vi "User_Database_Open.vi"(8 "error in (no error)":errorcluster caption="错误输入（无错误）", 11 "db Path":path=path "G:/2023项目/陆译电子/0008 User Management/Config/User_Info/User_Info.db") -> (0 "error out":errorcluster caption="错误输出", 3 "SQLite Connection":refnum<class "Connection.lvclass">)   [LabVIEW 2020]
uses:
  <vilib>/drjdpowell/SQLite Library/SQL Connection/Connection.lvclass
  <vilib>/drjdpowell/SQLite Library/SQL Connection/Open (path).vi
  <vilib>/drjdpowell/SQLite Library/SQL Connection/Open (string).vi
  <vilib>/AdvancedString/Path To Command Line String.vi
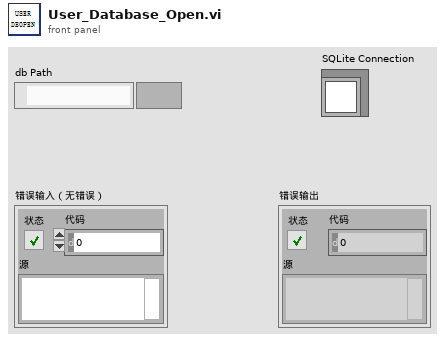
[diagram p1: front panel]
types:
  T1 = enum16{"New or existing", "Existing", "Read only"}
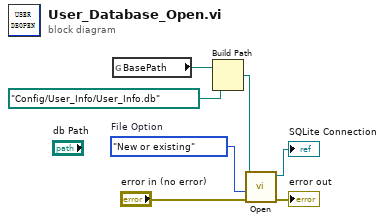
[diagram p0: block diagram]
diagram:
  w7 = T1."New or existing"  # File Option
  n1 = global read "Global.vi" "BasePath"() -> (w3:path)
  n2 = Build Path(base path=w3, name or relative path=path "Config/User_Info/User_Info.db") -> (appended path=w1:path)
  n3 = call-poly <vilib>:"Open.vi"("error in (no error)"="error in (no error)", "File Option"=w7, "db file"=w1) -> ("error out"=→"error out":errorcluster, "SQLite Connection"=→"SQLite Connection":refnum<class "Connection.lvclass">)  [unwired: 7 in]
